vi "Write Trace Level.vi"(8 "error in (no error)":errorcluster, 10 "Trace Level":T1(ring)=enum."Debug", 11 "Trace in":refnum<class "Trace.lvclass">) -> (0 "error out":errorcluster, 3 "Trace out":refnum<class "Trace.lvclass">)   [LabVIEW 2014, in "Robot Actor Framework.lvlib" / "Trace.lvlib" / "Trace.lvclass"]
uses:
  Trace.lvclass
  Trace.lvclass/Trace.ctl
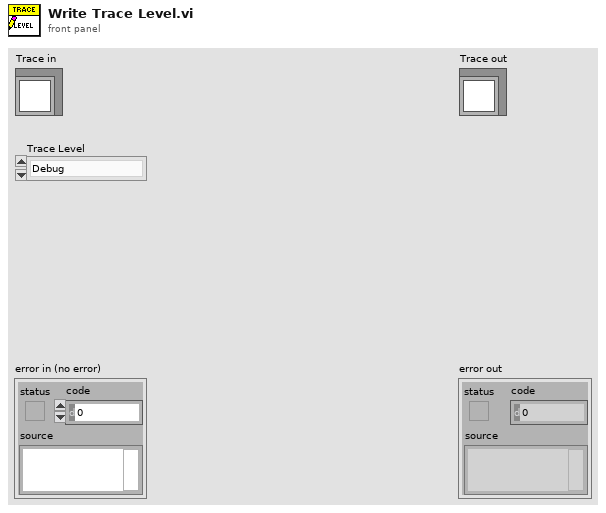
[diagram p1: front panel]
types:
  T1 = enum16{"Critical", "Error", "Warning", "Informational", "Debug"}
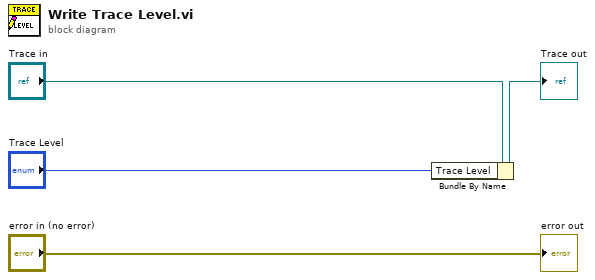
[diagram p0: block diagram]
diagram:
  n1 = Bundle By Name(cluster="Trace in", "Trace Level"="Trace Level") -> (→"Trace out":refnum<class "Trace.lvclass">)
  "error out" <- "error in (no error)"
